vi "poc.ip.vi"(0 "ip.reset":bool, 1 "TDATA":u64, 2 "TKEEP":u8, 3 "TUSER":bool, 4 "TVALID":bool, 5 "TLAST":bool) -> (14 "DEBUG.TDATA":u64, 15 "DEBUG.TKEEP":u8, 16 "DEBUG.TVALID":bool, 17 "DEBUG.TLAST":bool, 18 "command.valid":bool)   [LabVIEW 2020]
uses:
  submodules/Market.Data.Bats.Parser/fpga/poc.ip.debug.states.ctl
  <vilib>/Platform/TimedLoop/XDataNode/timing_clust.ctl
  <vilib>/Platform/TimedLoop/XDataNode/nitl_modes.ctl
  <vilib>/Platform/TimedLoop/XDataNode/wakeup.ctl
  <vilib>/rvi/Emulation/niFpgaSctlEmulationGetInTimedLoop.vi
  <vilib>/rvi/Emulation/niFpgaEmulationReportErrorSimple.vi
  <vilib>/rvi/Emulation/niFpgaGetClockAttributes.vi
  <vilib>/rvi/Emulation/niFpgaCriticalErrorInLSC.vi
  <vilib>/rvi/Emulation/niFpgaEmulationIsFPGAContextNoSignature.vi
  <vilib>/rvi/errors/niFpgaSetErrorForExecOnDevCompSimple.vi
  <vilib>/rvi/eio/common/nirviEmuReportErrorAndStop.vi
  <vilib>/rvi/DataTransferAndStorage/Container/Common/niFpgaContainerGetUniqueNameForEmu.vi
  <vilib>/rvi/FIFO/Fifo_Resource/nirvififoEmulationSetSize.vi
  <vilib>/rvi/FIFO/Fifo_Resource/nirviFifoEmulationQueueMgr.vi
  <instcachedir>/0/nirviFifoEmulationQueueMgr_E5CAEC123FF24DC58D834DCA3CDAA9B5.lvgen/nirviFifoEmulationQueueMgr_E5CAEC123FF24DC58D834DCA3CDAA9B5_008.vi
  <vilib>/Utility/error.llb/Clear Errors.vi
  <vilib>/rvi/FIFO/Fifo_Resource/nirvififoEmulationCreateLock.vi
  <vilib>/rvi/Emulation/niFpgaProcessEmulError.vi
  <vilib>/rvi/FIFO/Fifo_Resource/nirvififoEmulationObtainLock.vi
  <vilib>/rvi/FIFO/Fifo_Resource/nirvififoEmulationReleaseLock.vi
  <vilib>/rvi/occurrence/nirviWaitOnOccurrenceBase.vi
  <vilib>/rvi/errors/nirviReportUnexpectedCaseInternalError.vi
  <vilib>/rvi/errors/nirviReportUnexpectedCaseInternalError (U32).vi
  <instcachedir>/0/nirviFifoEmulationQueueMgr_E5CAEC123FF24DC58D834DCA3CDAA9B5.lvgen/nirviFifoEmulationQueueMgr_E5CAEC123FF24DC58D834DCA3CDAA9B5_020.vi
  <vilib>/Platform/TimedLoop/XDataNode/XDataNode.xnode
  <vilib>/rvi/DataTransferAndStorage/Container/XNode/niFpgaContainer.xnode
  <vilib>/rvi/FIFO/Fifo_Resource/nirvififoEmulationRead.vi
  <vilib>/Platform/TimedLoop/XDataNode/XDNodeRunTimeDep.lvlib
panel:
  out "command":T1
  # "This VI will be IP Exported"
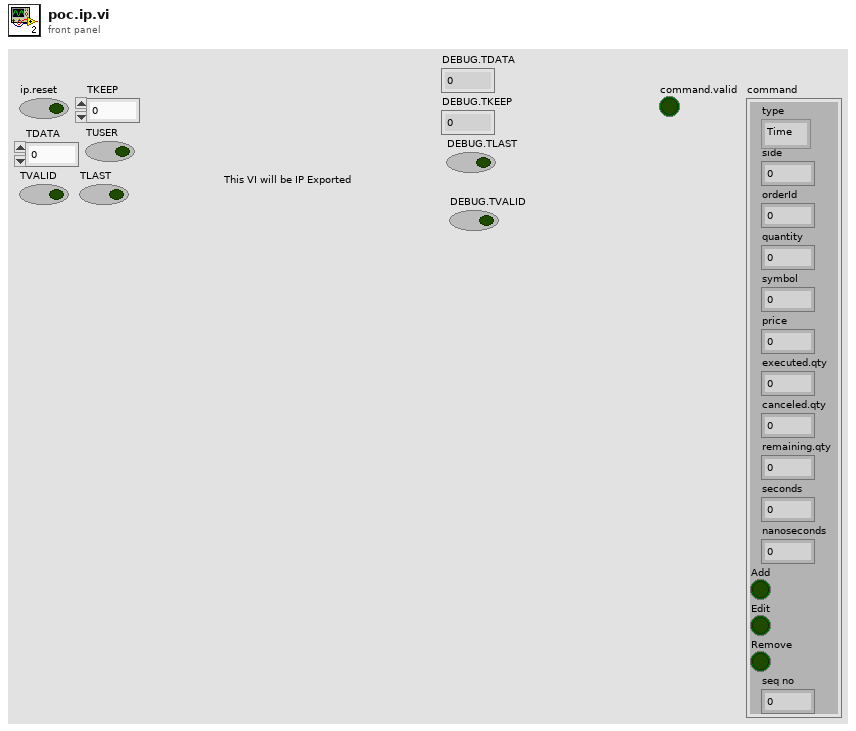
[diagram p1: front panel]
types:
  T1 = cluster{"type":enum8{"Time", "AddOrder", "OrderExecuted", "OrderExecutedAtPrice", "ReduceSize", "ModifyOrder", "DeleteOrder", "Get.Everything", "Get.All.Orders", "Get.Top"}, "side":u8, "orderId ":u64, "quantity":u32, "symbol":u64, "price":u64, "executed.qty":u32, "canceled.qty":u32, "remaining.qty":u32, "seconds":u64, "nanoseconds":u64, "Add":bool, "Edit":bool, "Remove":bool, "seq no":u32}
  T2 = typedef "poc.ip.debug.states.ctl" = enum16{"Wait.for.New.Packet", "Write.Data"}
  T3 = typedef "XDNodeRunTimeDep.lvlib/timing_clust.ctl" = cluster{"Expected End [f-1]":u64, "Actual End [f-1]":u64, "Finished Late? [f-1]":bool, "Expected End [i-1]":u64, "Actual End [i-1]":u64, "Finished Late? [i-1]":bool, "Expected Start [i]":u64, "Actual Start [i]":u64, "Expected Start [f]":u64, "Actual Start [f]":u64, "Source Name":string, "Structure Name":string, "Period":i64, "Deadline":i64, "Offset":i64, "Start":i64, "Priority":i32, "Timeout":i32, "Mode":T4, "Wakeup Reason":T5, "Error":errorcluster, "Source Type":string, "Secondary Source Type":string, "Global End Time":u64, "Global Start Time":u64, "Frame Duration":u64, "Iteration Duration":u64, "Assigned CPU":i32, "I/O Scan Engine Mode":u32}
  T4 = typedef "XDNodeRunTimeDep.lvlib/nitl_modes.ctl" = enum32{"No Change", "Process missed periods, maintain original phase", "Discard missed periods, maintain original phase", "Process missed periods, ignore original phase", "Discard missed periods, ignore original phase"}
  T5 = typedef "XDNodeRunTimeDep.lvlib/wakeup.ctl" = enum32{"Normal", "Aborted", "Asynchronous wakeup", "Timing source error", "Timed loop error", "Timeout"}
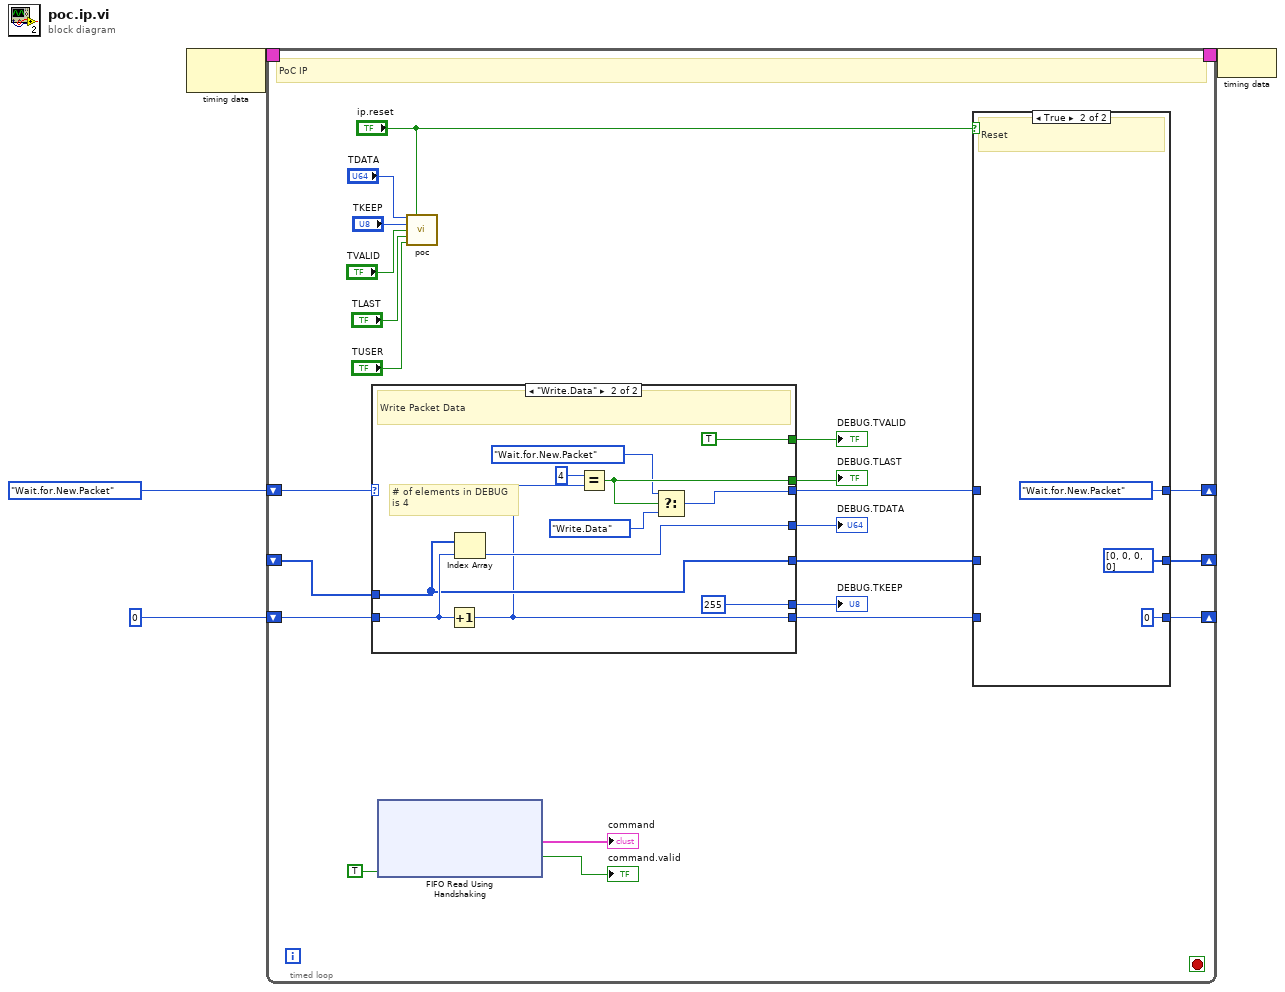
[diagram p0: block diagram]
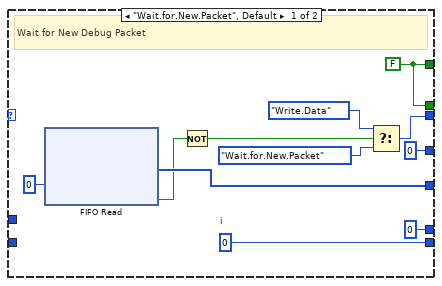
[diagram p3: hidden frame]
diagram:
  n1 = node-c288() -> (w4:T3)  [unwired: 1 in]
  n2 = timed-loop {
    timing: w4 -> [_]
    timing-out: [_] -> w3
    shift-right: [w16] -> _
    shift-left: poc.ip.debug.states."Wait.for.New.Packet" -> [w21]
    shift-right: [w19] -> _
    shift-left: i16 0 ("i") -> [w17]
    shift-right: [w13] -> _
    shift-left: _ -> [w12]
    stop <- _ stop-if-true
    # "PoC IP"
    n3 = case shown="\"Write.Data\"" w21 {
      tunnel: [w41 w49] -> w18
      tunnel: w17 -> [_ w54]
      tunnel: [w43 w46] -> w15
      tunnel: [w42 w53] -> w14
      tunnel: w12 -> [_ w53]
      tunnel: [u64 0 ("Data") w52] -> w11
      tunnel: [u8 0 ("DEBUG.TKEEP") u8 255 ("DEBUG.TKEEP")] -> w10
      tunnel: [w40 w47] -> w9
      tunnel: [w40 TRUE] -> w8
      frame "Wait.for.New.Packet", Default {
        w40 = FALSE
        w41 = i16 0  # i
        # "Wait for New Debug Packet"
        n4 = xnode "FIFO Read"("Timeout"=0) -> ("Element"=w42:u64[], "Timed Out?"=w33:bool)  [unwired: 1 in, 1 out]
        n5 = Not(x=w33) -> (.not. x?=w35:bool)
        n6 = Select(t=poc.ip.debug.states."Write.Data", s=w35, f=poc.ip.debug.states."Wait.for.New.Packet") -> (s? t:f=w43:T2)
      }
      frame "Write.Data" {
        # "# of elements in DEBUG\nis 4"
        # "Write Packet Data"
        n7 = Increment(x=w54) -> (x+1=w49:i16)
        n8 = Index Array(array=w53, index=w54) -> (element=w52:u64)
        n9 = Equal?(x=i16 4, y=w49) -> (x = y?=w47:bool)
        n10 = Select(t=poc.ip.debug.states."Wait.for.New.Packet", s=w47, f=poc.ip.debug.states."Write.Data") -> (s? t:f=w46:T2)
      }
    }
    "DEBUG.TDATA" <- w11
    "DEBUG.TKEEP" <- w10
    "DEBUG.TVALID" <- w8
    "DEBUG.TLAST" <- w9
    n11 = xnode "FIFO Read Using Handshaking"("Ready for Output"=TRUE) -> ("Element"=→"command":T1, "Output Valid"=→"command.valid":bool)  [unwired: 1 in, 1 out]
    n12 = call "poc.vi"("TDATA"="TDATA", "reset"="ip.reset", "TKEEP"="TKEEP", "TVALID"="TVALID", "TLAST"="TLAST", "TUSER"="TUSER") -> ()  [unwired: 10 in]
    n13 = case shown="True" "ip.reset" {
      tunnel: [w29 i16 0 ("i")] -> w19
      tunnel: w18 -> [w29 _]
      tunnel: [w28 poc.ip.debug.states."Wait.for.New.Packet"] -> w16
      tunnel: w15 -> [w28 _]
      tunnel: w14 -> [w27 _]
      tunnel: [w27 u64[] [0, 0, 0, 0] ("Element")] -> w13
      frame False {
        # "Pass Through"
      }
      frame True {
        # "Reset"
      }
    }
  }
  n14 = node-c288(w3) -> ()
